vi "GyroStream.vi"(8 "error in (no error)":errorcluster, 11 "connection ID":refnum<k16>) -> ()   [LabVIEW 2015]
uses:
  navx-mxp/labview/navX Library v2/navX Library v2.lvlib
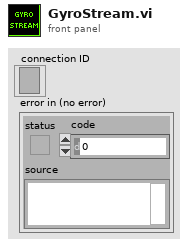
[diagram p1: front panel]
types:
  T1 = typedef "navX Library v2.lvlib/Z900_navX_DeviceTypeDef.ctl" = cluster{"Interface":cluster{"Protocol":T2, "Update Rate (4Hz-60Hz)":u8, "navX Open TypeDef":variant}, "Notify Packet":refnum<notifier>, "Loop VI Refnum":refnum<vi>, "Ready to Close Occurrence Refnum":refnum<k4>}
  T2 = typedef "navX Library v2.lvlib/Z900_navX_ProtocolTypeDef.ctl" = enum16{"SERIAL", "I2C", "SPI"}
  T3 = cluster{"Yaw":dbl, "Roll":dbl, "Pitch":dbl, "Heading":dbl, "Fused Heading":dbl}
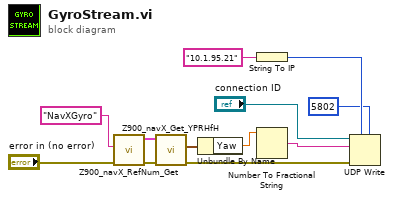
[diagram p0: block diagram]
diagram:
  n1 = call "Z900_navX_RefNum_Get.vi"("error in (no error)"="error in (no error)", "refnum name"="NavXGyro") -> ("error out"=w6:errorcluster, "navX Device"=w7:T1)  [unwired: 8 in]
  n2 = call "Z900_navX_Get_YPRHfH.vi"("error in (no error)"=w6, "navX Device"=w7) -> ("error out"=w2:errorcluster, "YRPHfH"=w4:T3)  [unwired: 6 in, 2 out]
  n3 = Unbundle By Name(w4) -> ("Yaw"=w1:dbl)
  n4 = String To IP(1:"10.1.95.21" ("name")) -> (0:w10:u32)
  n5 = Number To Fractional String(number=w1) -> (F-format string=w8:string)  [unwired: 3 in]
  n6 = UDP Write(address=w10, port or service name=u16 5802, connection ID="connection ID", data in=w8, 8:w2) -> ()  [unwired: 1 in, 2 out]
